vi "显示状态更新.vi"(9 "显示位数":u8=6 caption="显示位数(6)", 10 "码管数组引用":refnum<vi>, 11 "外观vi引用":refnum<vi>) -> ()   [LabVIEW 2013, in "数码管.xctl"]
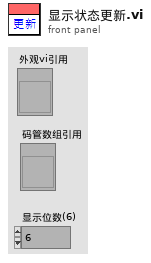
[diagram p1: front panel]
types:
  T1 = typedef "LVRectTypeDef.ctl" = cluster{"Left":i16, "Top":i16, "Right":i16, "Bottom":i16}
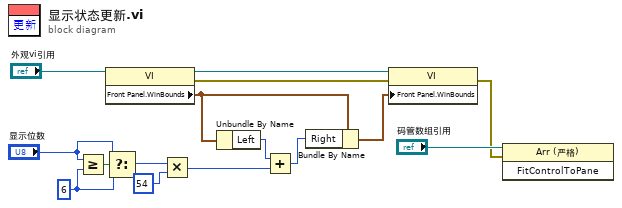
[diagram p0: block diagram]
diagram:
  w13 = u8 6 ("y")
  n1 = Greater Or Equal?(x="显示位数", y=w13) -> (x >= y?=w14:bool)
  n2 = property class="VI"(reference="外观vi引用") -> (reference out=w4:refnum<vi>, error out=w3:errorcluster, "Front Panel.WinBounds"=w9:T1)  [unwired: 1 in]
  n3 = Select(t="显示位数", s=w14, f=w13) -> (s? t:f=w11:u8)
  n4 = Multiply(x=w11, y=u8 54) -> (x*y=w8:u8)
  n5 = Unbundle By Name(w9) -> ("Left"=w7:i16)
  n6 = Add(x=w7, y=w8) -> (x+y=w6:i16)
  n7 = Bundle By Name(cluster=w9, "Right"=w6) -> (w5:T1)
  n8 = property class="VI"(reference=w4, error in=w3, "Front Panel.WinBounds"=w5) -> (error out=w1:errorcluster)  [unwired: 1 out]
  n9 = invoke class="Arr (严格)" method="FitControlToPane"(reference="码管数组引用", error in=w1) -> ()  [unwired: 1 in, 3 out]
